vi "_Read LC Inputs.vi"(1 "LogicOption":u8) -> (0 "LC Input Detected":bool)   [LabVIEW 2012]
uses:
  <vilib>/rvi/eio/common/nirviEmuTemplateMethod_errors.vi
  <vilib>/eio/EIONode/EIONode.xnode
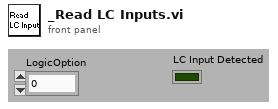
[diagram p1: front panel]
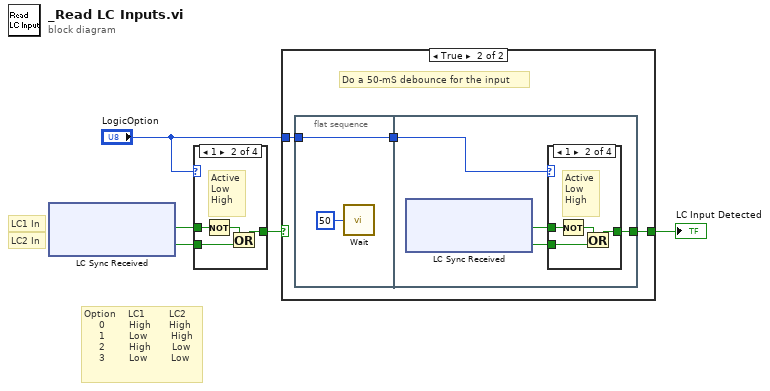
[diagram p0: block diagram]
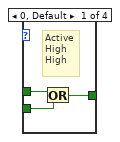
[diagram p2: hidden frame]
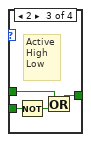
[diagram p3: hidden frame]
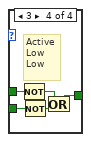
[diagram p4: hidden frame]
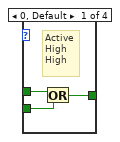
[diagram p6: hidden frame]
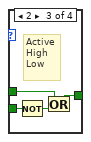
[diagram p7: hidden frame]
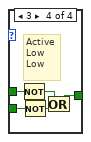
[diagram p8: hidden frame]
diagram:
  # "Option    LC1        LC2\n     0        High      High\n     1        Low        High\n     2        High       Low\n     3        Low        Low"
  # "LC2 In"
  # "LC1 In"
  n1 = xnode "LC Sync Received"() -> ("Digtal IO/DIO51"=w5:bool, "Digtal IO/DIO53"=w4:bool)  [unwired: 2 in, 2 out]
  n2 = case shown="1" "LogicOption" {
    tunnel: w5 -> [w8 w12 w13 w21]
    tunnel: w4 -> [w7 w9 w15 w20]
    tunnel: [w6 w10 w16 w17] -> w3
    frame 0, Default {
      # "Active\nHigh\nHigh"
      n3 = Or(x=w8, y=w7) -> (x .or. y?=w6:bool)
    }
    frame 1 {
      # "Active\nLow\nHigh"
      n4 = Not(x=w12) -> (.not. x?=w11:bool)
      n5 = Or(x=w11, y=w9) -> (x .or. y?=w10:bool)
    }
    frame 2 {
      # "Active\nHigh\nLow"
      n6 = Not(x=w15) -> (.not. x?=w14:bool)
      n7 = Or(x=w13, y=w14) -> (x .or. y?=w16:bool)
    }
    frame 3 {
      # "Active\nLow\nLow"
      n8 = Not(x=w21) -> (.not. x?=w18:bool)
      n9 = Not(x=w20) -> (.not. x?=w19:bool)
      n10 = Or(x=w18, y=w19) -> (x .or. y?=w17:bool)
    }
  }
  n11 = case shown="True" w3 {
    selector: w3 -> [w22 _]
    tunnel: [w22 w25] -> w2
    tunnel: "LogicOption" -> [_ w23]
    frame False {
    }
    frame True {
      # "Do a 50-mS debounce for the input"
      n12 = flat-sequence {
        tunnel: [w26] -> w24
        tunnel: w23 -> [w26]
        tunnel: [w31] -> w25
        tunnel: w24 -> [w28]
        frame #0 {
          n13 = call "Wait"("Count(mSec)"=u8 50) -> ()  [unwired: 1 out]
        }
        frame #1 {
          n14 = xnode "LC Sync Received"() -> ("Digtal IO/DIO51"=w30:bool, "Digtal IO/DIO53"=w29:bool)  [unwired: 2 in, 2 out]
          n15 = case shown="1" w28 {
            tunnel: w30 -> [w34 w38 w39 w47]
            tunnel: w29 -> [w33 w35 w41 w46]
            tunnel: [w32 w36 w42 w43] -> w31
            frame 0, Default {
              # "Active\nHigh\nHigh"
              n16 = Or(x=w34, y=w33) -> (x .or. y?=w32:bool)
            }
            frame 1 {
              # "Active\nLow\nHigh"
              n17 = Not(x=w38) -> (.not. x?=w37:bool)
              n18 = Or(x=w37, y=w35) -> (x .or. y?=w36:bool)
            }
            frame 2 {
              # "Active\nHigh\nLow"
              n19 = Not(x=w41) -> (.not. x?=w40:bool)
              n20 = Or(x=w39, y=w40) -> (x .or. y?=w42:bool)
            }
            frame 3 {
              # "Active\nLow\nLow"
              n21 = Not(x=w47) -> (.not. x?=w44:bool)
              n22 = Not(x=w46) -> (.not. x?=w45:bool)
              n23 = Or(x=w44, y=w45) -> (x .or. y?=w43:bool)
            }
          }
        }
      }
    }
  }
  "LC Input Detected" <- w2
